vi "create.messages.for.testing.vi"(11 "Messages to Create":T1[](array[typedef])) -> (3 "Words.Out":u16[](array[numeric]) format="%.0x")   [LabVIEW 2022 SP3]
uses:
  Message.Spec.ctl
  pitch/MessageType.ctl
  pitch/AddOrderLong/AddOrderLong.Parameters.ctl
  pitch/Time/Time.Parameters.ctl
  pitch/SequencedUnitHeader/SequencedUnitHeader.Parameters.ctl
  pitch/SequencedUnitHeader/SequencedUnitHeader.lvclass
  pitch/Time/Time.lvclass
  pitch/AddOrderLong/AddOrderLong.lvclass
panel:
  out "size(s)":i32
  out "Remaining Bytes":u8[](array[numeric])
  out "Raw.Bytes.Out":u8[](array[numeric]) format="%.0x"
  out "Bytes.out (Visual)":u8[][](array[numeric]) format="%.0x"
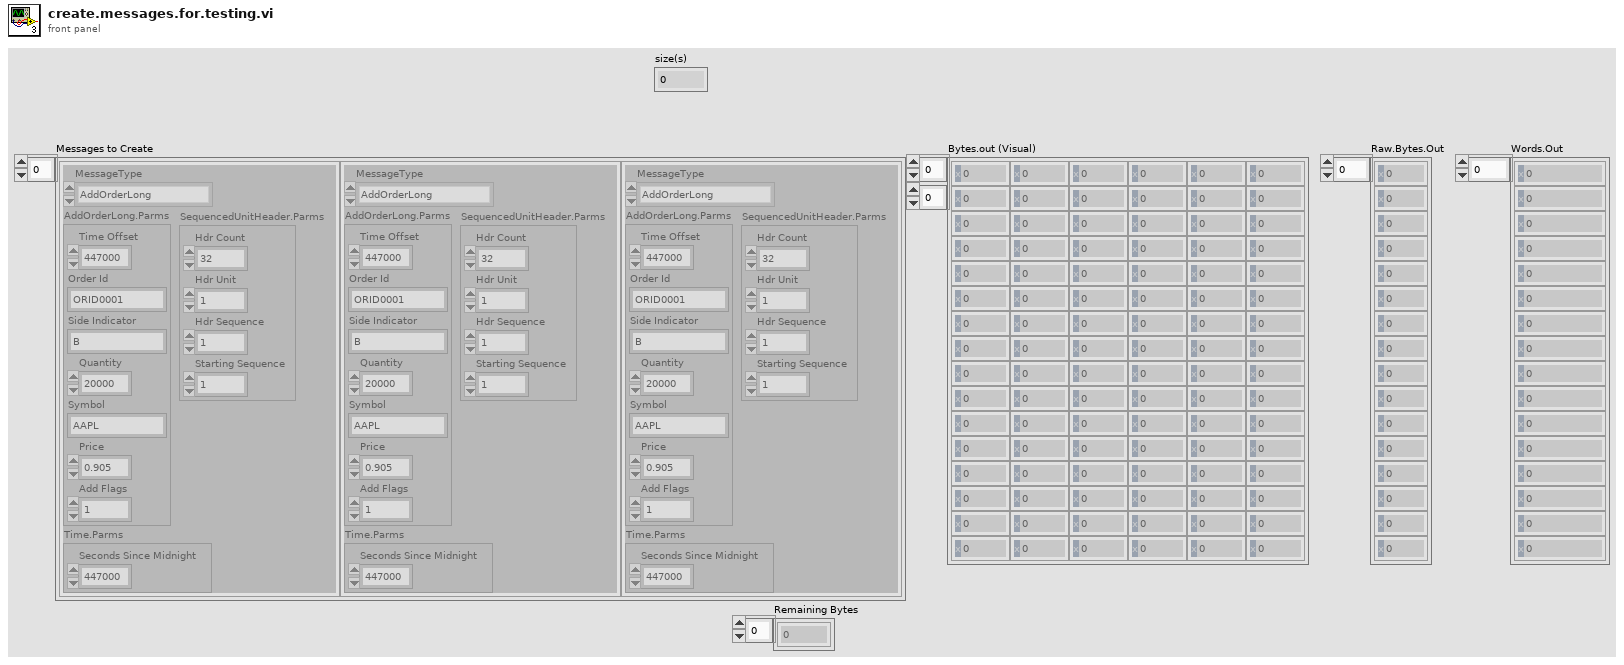
[diagram p1: front panel]
types:
  T1 = typedef "Message.Spec.ctl" = cluster{"MessageType":T2, "AddOrderLong.Parms":T3, "Time.Parms":T4, "SequencedUnitHeader.Parms":T5}
  T2 = typedef "MessageType.ctl" = enum16{"SequencedUnitHeader", "AddOrderLong", "AddOrderShort", "AddOrderExpanded", "Time"}
  T3 = typedef "AddOrderLong.lvclass/AddOrderLong.Parameters.ctl" = cluster{"Time Offset":u32, "Order Id":string, "Side Indicator":string, "Quantity":u32, "Symbol":string, "Price":dbl, "Add Flags":u8}
  T4 = typedef "Time.lvclass/Time.Parameters.ctl" = cluster{"Seconds Since Midnight":u32}
  T5 = typedef "SequencedUnitHeader.lvclass/SequencedUnitHeader.Parameters.ctl" = cluster{"Hdr Count":u8, "Hdr Unit":u8, "Hdr Sequence":u32, "Starting Sequence":u32}
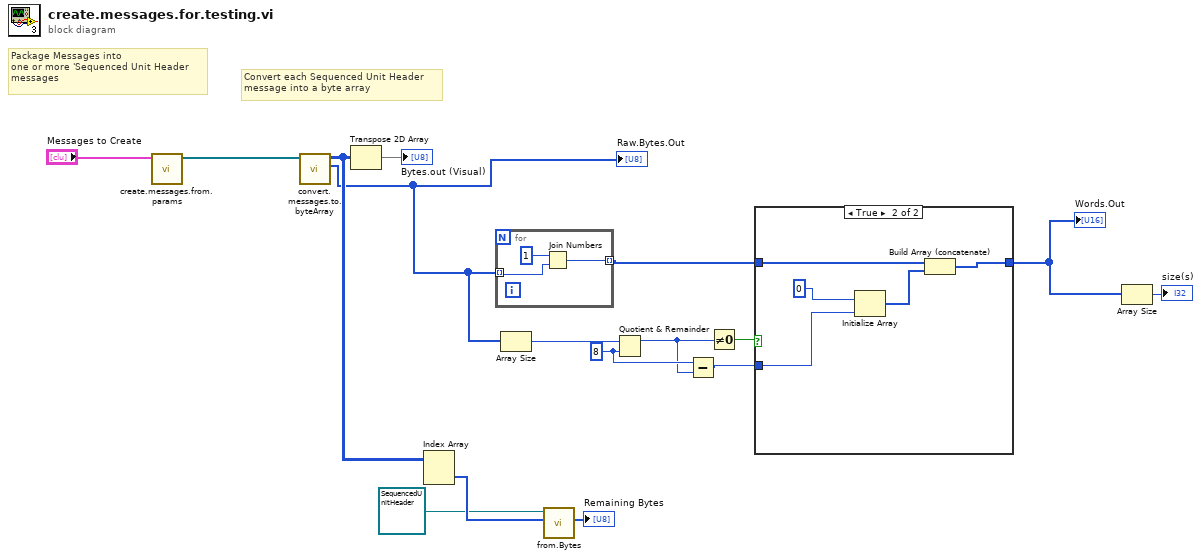
[diagram p0: block diagram]
diagram:
  w7 = 8 ("y")
  # "Convert each Sequenced Unit Header\nmessage into a byte array"
  # "Package Messages into\none or more 'Sequenced Unit Header\nmessages"
  n1 = call "create.messages.from.params.vi"("Messages to Create"="Messages to Create") -> ("Messages.Out"=w15:refnum<class "SequencedUnitHeader.lvclass">[])  [unwired: 10 in]
  n2 = call "convert.messages.to.byteArray.vi"("Messages.In"=w15) -> ("ByteArray.out"=w8:u8[], "2D.ByteArray.out"=w10:u8[][])  [unwired: 9 in]
  "Raw.Bytes.Out" <- w8
  n3 = Transpose 2D Array(2D array=w10) -> (transposed array=→"Bytes.out (Visual)":u8[][])
  n4 = Index Array(array=w10) -> (element=w13:u8[])  [unwired: 2 in]
  n5 = for {
    tunnel: w8 -> [w19] mode=indexing
    tunnel: [w17] -> w4 mode=indexing
    n6 = Join Numbers(hi=u8 1, lo=w19) -> ((hi.lo)=w17:u16)
  }
  n7 = Array Size(array=w8) -> (size(s)=w9:i32)
  n8 = call-dynamic "from.Bytes.vi"("Bytes.In"=w13, "SequencedUnitHeader in"=refnum<class "SequencedUnitHeader.lvclass"> refnum ("SequencedUnitHeader.lvclass")) -> ("Remaining Bytes"=→"Remaining Bytes":u8[])  [unwired: 7 in, 2 out]
  n9 = Quotient & Remainder(x=w9, y=w7) -> (x-y*floor(x/y)=w6:i32)  [unwired: 1 out]
  n10 = Subtract(x=w7, y=w6) -> (x-y=w3:i32)
  n11 = Not Equal To 0?(x=w6) -> (x != 0?=w5:bool)
  n12 = case shown="True" w5 {
    tunnel: w4 -> [w20 w24]
    tunnel: [w20 w23] -> w2
    tunnel: w3 -> [_ w21]
    frame False {
    }
    frame True {
      n13 = Initialize Array(u16 0, w21) -> (w25:u16[])
      n14 = Build Array (concatenate)(w24, w25) -> (w23:u16[])
    }
  }
  "Words.Out" <- w2
  n15 = Array Size(array=w2) -> (size(s)=→"size(s)":i32)
